vi "Main (RT).vi"() -> ()   [LabVIEW 2015]
uses:
  <vilib>/FPGAPlugInAG/myRIO-1900/niLvFpga_Open_myRIO-1900.vi
  <vilib>/Utility/error.llb/Error Cluster From Error Code.vi
  <vilib>/rvi/errors/niLvFpgaAdjustHostInterfaceError.vi
  <vilib>/FPGAPlugInAG/myRIO-1900/niLvFpga_Close_myRIO-1900.vi
  <vilib>/addons/Fuzzy Logic/FL Fuzzy Controller (MISO).vi
  <vilib>/Utility/file.llb/Write Delimited Spreadsheet (string).vi
  <vilib>/rvi/interface/common/dynamic/niFpgaDynamicAddResources.vi
  <vilib>/FPGAPlugInAG/Dynamic/niLvFpga_Close_Dynamic.vi
  <vilib>/rvi/interface/nirviOpenFPGA/nirviOpenFPGA.xnode
  FPGA Bitfiles/DHT11Sensor_FPGATarget_[FPGA]Main2_3IYteBULfXM.lvbitx
  DHT11 Library/Example - DHT11 (FPGA).vi
  <vilib>/rvi/interface/nirviReadWriteControl/nirviReadWriteControl.xnode
  <vilib>/rvi/interface/nirviCloseFPGA/nirviCloseFPGA.xnode
  FPGA Bitfiles/DHT11Sensor_FPGATarget_cobaaa3_ag5UYFczPYI.lvbitx
  C:/Users/ririn/Documents/LabVIEW Data/ririn/cobaaa.vi
  FPGA Bitfiles/DHT11Sensor_FPGATarget_cobat2_iTASjCldgZM.lvbitx
  C:/Users/ririn/Documents/LabVIEW Data/ririn/cobat.vi
  <vilib>/addons/Fuzzy Logic/NI_Fuzzy_Logic_API.lvlib
  <vilib>/rvi/interface/Simulation/niFpgaSimulationCallBeginRW.vi
  NiFpgaLv.dll
panel:
  in  "stop 5":bool
  in  "stop 4":bool
  in  "stop":bool
  in  "Tab Control 2":T1(tab)
  out "Humidity (%)":dbl
  out "Temperature (C)":dbl
  out "Open AC":dbl(slide) scale=0.0..35.0
  out "Tidak Nyaman":bool
  out "Nyaman":bool
  in  "Stop 3":bool
  out "Nilai Fuzzy Logic Control":dbl
  out "Temperature (°C)":u8
  out "Humidity (%)":u8
  in  "MAX  3":dbl
  in  "MIN   1":dbl
  in  "MAX   7":dbl
  in  "MIN   8":dbl
  in  "stop":bool
  in  "Data Manual":bool
  in  "Temperature (C)":dbl
  in  "Humidity (%)  2":dbl
  out "Temperature (C) 2":dbl(slide) scale=0.0..50.0
  out "Humidity (%)  3":dbl(slide) scale=0.0..90.0
  in  "Temperature C":dbl
  in  "Humidity %":dbl
  out "Humidity (%)  4":dbl(slide) scale=0.0..90.0
  out "Temperature (C)3":dbl(slide) scale=0.0..50.0
  in  "MIN   2":dbl
  in  "MAX  2":dbl
  out "Cukup Nyaman":bool
  in  "View":bool
  in  "data":string[][](table)
  in  "SAVE":bool
  out "Data":string
  in  "Restart":bool
  # "SISTEM KONTROL DAN MONITORING AIR CONDITIONER ( AC )"
  # "Aturan Penggunaan :\n\n1. Di dalam interface sistem ini terdapat 3 halaman yaitu Aturan Penggunaan, Control System dan Monitor Data Sensor, dimana masing-masing halaman memiliki   fungsi yang berbeda-beda. jika ingin melihat dari masing-masing halaman user dapat mengklik tab-tab yang ada di pajok kiri atas yang terdapat nama dari masing-masing halaman. \n  \n2. Sebelum mengaktifkan sistem ini, user harus memasukkan nilai minimal dan maksimal kondisi ruangan yang telah ditetapkan yang terdapat pada halaman Control System, akan tetapi jika user inggin menganti nilai standarnya kondisi ruangan user dapat melakukan analisa untuk mendapatkan nilai yang diinginkan.\n\n3.  Setelah user mengaktifkan sistem, jika ingin melakukan pengecekan pada sistem maka user dapat mengaktifkan data manual dengan cara mengaktifkan saklar ON, setelah itu user dapat memberi data input sesuai keinginan user. (catatan : jika data manual aktif maka data sensor akan mati).\n\n4. User dapat memonitoring dan menyimpan data sensor dihalaman Monitor Data Sensor, jika ingin menyimpan data sensor maka user cukup mengklik 1 x tombol Save, maka data akan tersimpan didalam memory myRIO. dan jika user ingin menampilkan kembali data yang sudah disimpan maka user cukup klik tombol View. (catatan : jika data yang ditampilkan tidak sesuai maka sistem dapat direstart dengang mengkil 1x tombol Restart)"
  # "sensors"
  # "Fuzzy\nController"
  # "actuators"
  # "Kondisi Ruangan"
  # "INDICATOR DATA INPUT"
  # "Nilai standart untuk kondisi Ruangan adalah :\nJika Tidak Ada Standart sensiri isi sesuai Dibawah ini !!!\n(PANAS)\nuntuk Ststus Tidak Nyaman MIN [8] MAX [20]\n(SEJUK)\nuntuk Status Nyaman MIN [20] MAX [26]\n(DINGIN)\nuntuk Status Cukup Nyaman MIN [26] MAX [35]"
  # "Temperature (C)"
  # "Humidity (%)"
  # "Indikator Kondisi Ruangan"
  # "DATA MANUAL"
  # "INDICATOR DATA SENSOR"
  # "ON"
  # "OFF"
  # "Date"
  # "Time"
  # "Temperature (C)"
  # "Humidity (%)"
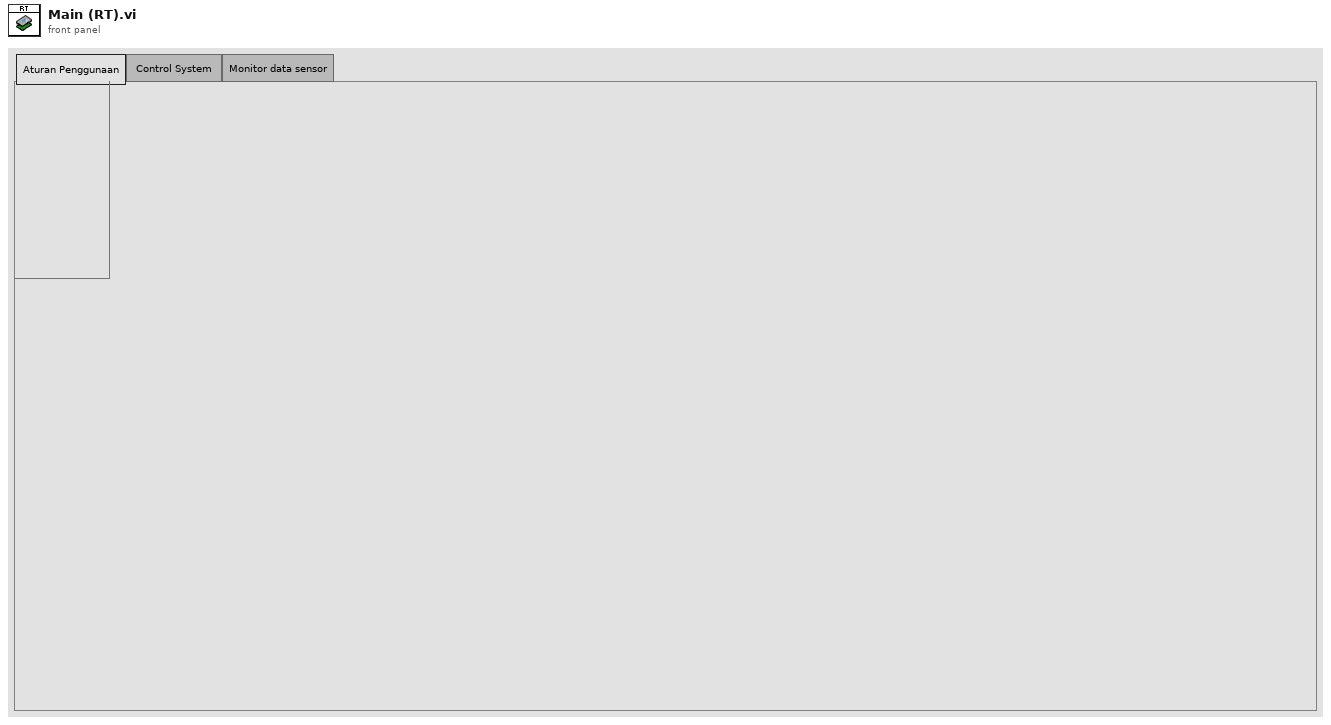
[diagram p1: front panel]
types:
  T1 = enum32{"Aturan Penggunaan", "Control System  ", "Monitor data sensor"}
  T2 = enum16{"open", "replace", "create", "open or create", "replace or create", "replace or create with confirmation"}
  T3 = typedef "NI_Fuzzy_Logic_API.lvlib/FL System.ctl" = cluster{"input variables":T4[], "output variables":T4[], "rules":T7[], "defuzzification method":T13, "description":string, "user MF interpolating polynomials":T14[]}
  T4 = typedef "NI_Fuzzy_Logic_API.lvlib/FL Variable.ctl" = cluster{"name":string, "range":dbl[], "MFs":T5[]}
  T5 = typedef "NI_Fuzzy_Logic_API.lvlib/FL Membership Function.ctl" = cluster{"name":string, "shape":T6, "points":dbl[], "color":u32, "user-defined shape index":i32}
  T6 = typedef "NI_Fuzzy_Logic_API.lvlib/FL Membership Function Shape.ctl" = u16
  T7 = typedef "NI_Fuzzy_Logic_API.lvlib/FL Rule.ctl" = cluster{"antecedents":T8[], "antecedent connective":T10, "consequents":T11[], "consequent implication":T12, "degree of support":dbl}
  T8 = typedef "NI_Fuzzy_Logic_API.lvlib/FL Antecedent.ctl" = cluster{"Var Index":i32, "MF Index":i32, "Cond":T9}
  T9 = typedef "NI_Fuzzy_Logic_API.lvlib/FL Modifier.ctl" = u16
  T10 = typedef "NI_Fuzzy_Logic_API.lvlib/FL Antecedent Connective.ctl" = u16
  T11 = typedef "NI_Fuzzy_Logic_API.lvlib/FL Consequent.ctl" = cluster{"Var Index":i32, "MF Index":i32, "Cond":T9}
  T12 = typedef "NI_Fuzzy_Logic_API.lvlib/FL Consequent Implication.ctl" = u16
  T13 = typedef "NI_Fuzzy_Logic_API.lvlib/FL Defuzzification.ctl" = u16
  T14 = typedef "NI_Fuzzy_Logic_API.lvlib/FL Interpolating polynomials.ctl" = cluster{"X":dbl[], "Y":dbl[], "Y(x) coeff":dbl[][], "X(y) coeff":dbl[][], "Area(y) coeff":dbl[][], "coa_x(y) coeff":dbl[][]}
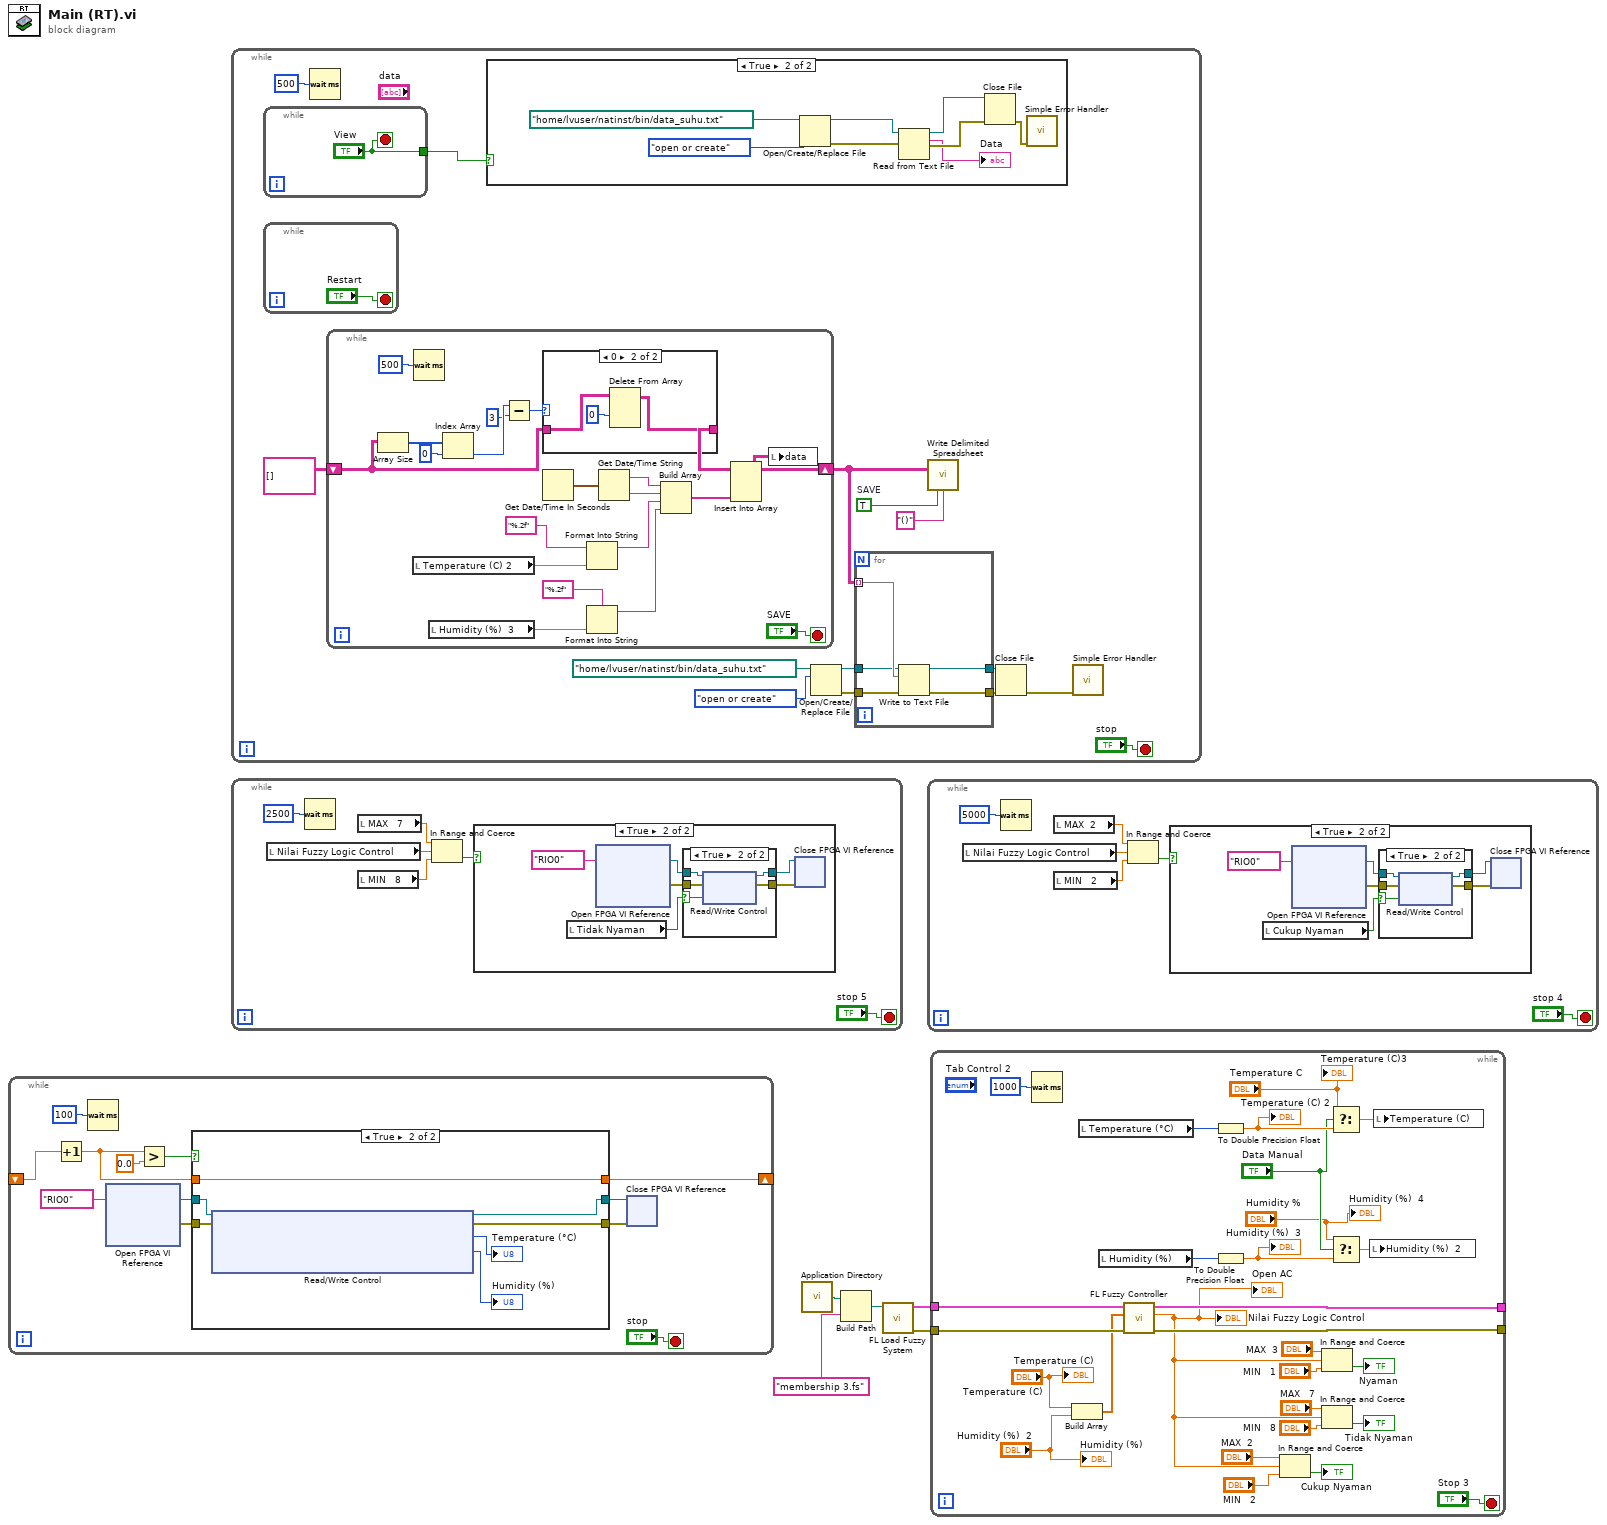
[diagram p0: block diagram]
diagram:
  n1 = while {
    shift-right: [w12] -> _
    shift-left: _ -> [w11]
    stop <- "stop" stop-if-true
    n2 = Increment(x=w11) -> (x+1=w7:dbl)
    n3 = Wait (ms)(milliseconds to wait=u32 100) -> ()  [unwired: 1 out]
    n4 = xnode "Open FPGA VI Reference"("resource name"=tag "RIO0") -> ("FPGA VI Reference Out"=w16:refnum<k20>, "error out"=w17:errorcluster)  [unwired: 1 in]
    n5 = Greater?(x=w7, y=0.0) -> (0:w9:bool)
    n6 = case shown="True" w9 {
      tunnel: [_ w24] -> w13
      tunnel: [_ w23] -> w14
      tunnel: w16 -> [_ w22]
      tunnel: w17 -> [_ w21]
      tunnel: [_ w20] -> w12
      tunnel: w7 -> [_ w20]
      frame False {
      }
      frame True {
        n7 = xnode "Read/Write Control"("FPGA VI Reference In"=w22, "error in"=w21) -> ("FPGA VI Reference Out"=w24:refnum<k20>, "error out"=w23:errorcluster, "Temperature (°C)"=→"Temperature (°C)":u8, "Humidity (%)"=→"Humidity (%)":u8)  [unwired: 1 out]
      }
    }
    n8 = xnode "Close FPGA VI Reference"("FPGA VI Reference In"=w13, "error in"=w14) -> ()  [unwired: 1 out]
  }
  n9 = while {
    stop <- "stop" stop-if-true
    w38 = TRUE  # SAVE
    n10 = while {
      tunnel: ["View"] -> w25
      stop <- "View" stop-if-true
    }
    n11 = while {
      stop <- "Restart" stop-if-true
    }
    n12 = Wait (ms)(milliseconds to wait=u32 500) -> ()  [unwired: 1 out]
    n13 = while {
      shift-right: [w55] -> w26
      shift-left: string[][] [] -> [w58]
      stop <- "SAVE" stop-if-true
      n14 = Array Size(array=w58) -> (size(s)=w66:i32[])
      n15 = local read "Temperature (C) 2"() -> (w60:dbl)
      n16 = Wait (ms)(milliseconds to wait=u32 500) -> ()  [unwired: 1 out]
      n17 = local read "Humidity (%)  3"() -> (w59:dbl)
      n18 = Index Array "Index Array"(array=w66, index=0) -> (element=w64:i32)
      n19 = Subtract(x=w64, y=3) -> (x-y=w62:i32)
      n20 = case shown="0" w62 {
        tunnel: w58 -> [w74 w77]
        tunnel: [w74 w76] -> w56
        frame Default {
        }
        frame 0 {
          n21 = Delete From Array "Delete From Array"(array=w77, index (row)=0) -> (array with subset deleted=w76:string[][])  [unwired: 2 in, 1 out]
        }
      }
      n22 = Get Date/Time In Seconds() -> (seconds since 1Jan1904=w67:timestamp)
      n23 = Format Into String "Format Into String"(format string="%.2f", w60) -> (resulting string=w71:string)  [unwired: 2 in, 1 out]
      n24 = Format Into String(format string="%.2f", w59) -> (resulting string=w70:string)  [unwired: 2 in, 1 out]
      n25 = Get Date/Time String(seconds (now)=w67) -> (date string=w69:string, time string=w68:string)  [unwired: 2 in]
      n26 = Build Array "Build Array"(w69, w68, w71, w70) -> (w61:string[])
      n27 = Insert Into Array "Insert Into Array"(array=w56, new element=w61) -> (w55:string[][])  [unwired: 2 in]
      n28 = local write "data"(w55) -> ()
    }
    n29 = case shown="True" w25 {
      frame False {
      }
      frame True {
        n30 = Open/Create/Replace File(file path (use dialog)=path "/home/lvuser/natinst/bin/data_suhu.txt", operation (0:open)=T2."open or create") -> (refnum out=w45:refnum<file>, error out=w46:errorcluster)  [unwired: 4 in, 1 out]
        n31 = Read from Text File(file (use dialog)=w45, error in=w46) -> (refnum out=w47:refnum<file>, text=→"Data":string, error out=w48:errorcluster)  [unwired: 2 in, 1 out]
        n32 = Close File(refnum=w47, error in=w48) -> (error out=w44:errorcluster)  [unwired: 1 out]
        n33 = call <vilib>:"Simple Error Handler.vi"("error in (no error)"=w44) -> ()  [unwired: 4 in, 5 out]
      }
    }
    n34 = Open/Create/Replace File(file path (use dialog)=path "/home/lvuser/natinst/bin/data_suhu.txt", operation (0:open)=T2."open or create") -> (refnum out=w30:refnum<file>, error out=w31:errorcluster)  [unwired: 4 in, 1 out]
    n35 = for {
      tunnel: w26 -> [w53] mode=indexing
      tunnel: w30 -> [w52]
      tunnel: w31 -> [w51]
      tunnel: [w50] -> w32
      tunnel: [w49] -> w33
      n36 = Write to Text File(file (use dialog)=w52, text=w53, error in=w51) -> (refnum out=w50:refnum<file>, error out=w49:errorcluster)  [unwired: 1 in, 1 out]
    }
    n37 = call-poly <vilib>:"Write Delimited Spreadsheet.vi"("2D data"=w26, "transpose? (F)"=w38, "delimiter (\\t)"="()" ("delimiter (\\t)")) -> ()  [unwired: 11 in, 2 out]
    n38 = Close File(refnum=w32, error in=w33) -> (error out=w29:errorcluster)  [unwired: 1 out]
    n39 = call <vilib>:"Simple Error Handler.vi"("error in (no error)"=w29) -> ()  [unwired: 4 in, 5 out]
  }
  n40 = while {
    stop <- "stop 5" stop-if-true
    n41 = local read "Nilai Fuzzy Logic Control"() -> (w82:dbl)
    n42 = Wait (ms)(milliseconds to wait=u32 2500) -> ()  [unwired: 1 out]
    n43 = local read "MAX   7"() -> (w81:dbl)
    n44 = local read "MIN   8"() -> (w80:dbl)
    n45 = In Range and Coerce(upper limit=w81, x=w82, lower limit=w80) -> (In Range?=w83:bool)  [unwired: 1 out]
    n46 = case shown="True" w83 {
      frame False {
      }
      frame True {
        n47 = local read "Tidak Nyaman"() -> (w87:bool)
        n48 = xnode "Open FPGA VI Reference"("resource name"=tag "RIO0") -> ("FPGA VI Reference Out"=w86:refnum<k20>, "error out"=w85:errorcluster)  [unwired: 1 in]
        n49 = case shown="True" w87 {
          selector: w87 -> [_ w90]
          tunnel: w86 -> [_ w94]
          tunnel: w85 -> [_ w93]
          tunnel: [_ w92] -> w89
          tunnel: [_ w91] -> w88
          frame False {
          }
          frame True {
            n50 = xnode "Read/Write Control"("FPGA VI Reference In"=w94, "error in"=w93, "LED 2"=w90) -> ("FPGA VI Reference Out"=w92:refnum<k20>, "error out"=w91:errorcluster)
          }
        }
        n51 = xnode "Close FPGA VI Reference"("FPGA VI Reference In"=w89, "error in"=w88) -> ()  [unwired: 1 out]
      }
    }
  }
  n52 = call <vilib>:"Application Directory.vi"() -> ("Application Directory"=w4:path)
  n53 = Build Path(base path=w4, name or relative path="membership 3.fs") -> (appended path=w3:path)
  n54 = call <vilib>:"FL Load Fuzzy System.vi"("file path"=w3) -> ("error out"=w1:errorcluster, "fuzzy system out"=w2:T3)  [unwired: 1 in, 8 out]
  n55 = while {
    stop <- "stop 4" stop-if-true
    n56 = local read "Nilai Fuzzy Logic Control"() -> (w99:dbl)
    n57 = Wait (ms)(milliseconds to wait=u32 5000) -> ()  [unwired: 1 out]
    n58 = local read "MAX  2"() -> (w98:dbl)
    n59 = local read "MIN   2"() -> (w97:dbl)
    n60 = In Range and Coerce(upper limit=w98, x=w99, lower limit=w97) -> (In Range?=w100:bool)  [unwired: 1 out]
    n61 = case shown="True" w100 {
      frame False {
      }
      frame True {
        n62 = local read "Cukup Nyaman"() -> (w101:bool)
        n63 = xnode "Open FPGA VI Reference"("resource name"=tag "RIO0") -> ("FPGA VI Reference Out"=w105:refnum<k20>, "error out"=w104:errorcluster)  [unwired: 1 in]
        n64 = case shown="True" w101 {
          selector: w101 -> [_ w107]
          tunnel: w105 -> [_ w111]
          tunnel: w104 -> [_ w110]
          tunnel: [_ w109] -> w103
          tunnel: [_ w108] -> w102
          frame False {
          }
          frame True {
            n65 = xnode "Read/Write Control"("FPGA VI Reference In"=w111, "error in"=w110, "LED"=w107) -> ("FPGA VI Reference Out"=w109:refnum<k20>, "error out"=w108:errorcluster)
          }
        }
        n66 = xnode "Close FPGA VI Reference"("FPGA VI Reference In"=w103, "error in"=w102) -> ()  [unwired: 1 out]
      }
    }
  }
  n67 = while {
    tunnel: [w137] -> _
    tunnel: [w136] -> _
    tunnel: w2 -> [w135]
    tunnel: w1 -> [w134]
    stop <- "Stop 3" stop-if-true
    n68 = Wait (ms)(milliseconds to wait=u32 1000) -> ()  [unwired: 1 out]
    n69 = Build Array "Build Array"("Temperature (C)", "Humidity (%)  2") -> (w131:dbl[])
    n70 = local read "Temperature (°C)"() -> (w127:u8)
    n71 = local read "Humidity (%)"() -> (w126:u8)
    n72 = call-poly <vilib>:"FL Fuzzy Controller.vi"("error in (no error)"=w134, "input values"=w131, "fuzzy system in"=w135) -> ("error out"=w136:errorcluster, "output value"=w116:dbl, "fuzzy system out"=w137:T3)  [unwired: 6 out]
    "Nilai Fuzzy Logic Control" <- w116
    "Open AC" <- w116
    n73 = To Double Precision Float(number=w127) -> (double precision float=w122:dbl)
    "Temperature (C) 2" <- w122
    n74 = To Double Precision Float(number=w126) -> (double precision float=w123:dbl)
    "Humidity (%)  3" <- w123
    n75 = In Range and Coerce(upper limit="MAX  2", x=w116, lower limit="MIN   2") -> (In Range?=→"Cukup Nyaman":bool)  [unwired: 1 out]
    n76 = In Range and Coerce(upper limit="MAX  3", x=w116, lower limit="MIN   1") -> (In Range?=→"Nyaman":bool)  [unwired: 1 out]
    n77 = In Range and Coerce(upper limit="MAX   7", x=w116, lower limit="MIN   8") -> (In Range?=→"Tidak Nyaman":bool)  [unwired: 1 out]
    n78 = Select(t="Temperature C", s="Data Manual", f=w122) -> (s? t:f=w125:dbl)
    n79 = Select(t="Humidity %", s="Data Manual", f=w123) -> (s? t:f=w124:dbl)
    n80 = local write "Humidity (%)  2"(w124) -> ()
    n81 = local write "Temperature (C)"(w125) -> ()
    "Humidity (%)" <- "Humidity (%)  2"
    "Temperature (C)" <- "Temperature (C)"
    "Temperature (C)3" <- "Temperature C"
    "Humidity (%)  4" <- "Humidity %"
  }
